vi "fetch frame usb 悉灵.vi"() -> ()   [LabVIEW 2015]
uses:
  <vilib>/Utility/miscctls.llb/LV3DPointTypeDef.ctl
  <vilib>/Utility/miscctls.llb/LVRGBAColorTypeDef.ctl
  <userlib>/Mv3dRgbd/Mv3dRgbd.lvlib
  <vilib>/picture/3D Picture Control/NI_3D Picture Control.lvlib
  <userlib>/Mv3dRgbdEx/Mv3dRgbdEx.lvlib
panel:
  out "handle out 4":u32
  out "pProcess out":u32
  out "function return 6":i32
  in  "pProcess":u32
  out "handle out 3":u32
  out "function return 5":i32
  out "pstParam out":T1={"enParamType"=1, "nReserved[0]"=0, "nReserved[1]"=0, "nReserved[2]"=0, "nReserved[3]"=0, "nReserved[4]"=0, "nReserved[5]"=0, "nReserved[6]"=0, "nReserved[7]"=0, "nReserved[8]"=0, "nReserved[9]"=0, "nReserved[10]"=0, "nReserved[11]"=0, "nReserved[12]"=0, "nReserved[13]"=0, "nReserved[14]"=0, "nReserved[15]"=0} {"enParamType" items=["ParamType_Bool"=1, "ParamType_Int"=2, "ParamType_Float"=3, "ParamType_Enum"=4, "ParamType_String"=5]}
  in  "strKey":string
  in  "pstParam":T1={"enParamType"=1, "nReserved[0]"=0, "nReserved[1]"=0, "nReserved[2]"=0, "nReserved[3]"=0, "nReserved[4]"=0, "nReserved[5]"=0, "nReserved[6]"=0, "nReserved[7]"=0, "nReserved[8]"=0, "nReserved[9]"=0, "nReserved[10]"=0, "nReserved[11]"=0, "nReserved[12]"=0, "nReserved[13]"=0, "nReserved[14]"=0, "nReserved[15]"=0} {"enParamType" items=["ParamType_Bool"=1, "ParamType_Int"=2, "ParamType_Float"=3, "ParamType_Enum"=4, "ParamType_String"=5]}
  out "function return 4":i32
  out "pDeviceNumber out":u32
  in  "pDeviceNumber":u32
  out "handle out":u32
  out "function return 3":i32
  out "pstCalibInfo out":T2
  in  "nCoordinateType":u32
  in  "pstCalibInfo":T2
  out "function return 2":i32
  out "size 3":i32
  out "address 3":i64
  out "pYuvImgge out":T3
  in  "handle":u32
  out "pstU3DeviceInfo out":T4
  out "function return":i32
  out "get list return":i32
  out "pDeviceCount out 2":u32
  out "address 2":i64
  out "size 4":i32
  out "address 5":i64
  in  "?":enum32{"RGBD", "点云"}(tab)
  out "Depth":i16[][](graph)
  out "RGB":picture
  out "start function":i32
  out "stop function":i32
  out "release function":i32
  out "init function":i32
  out "close function":i32
  in  "?":bool
  out "fetchframe function":i32
  out "depthtocloud return":i32
  out "yuv422torgb return":i32
  out "MV3D_RGBD_GigEDEVICE_INFO out 3":T5(array[cluster])
  out "?":refnum<vi>(3d-picture)
  in  "Character Size":sgl=0.5 caption="字符大小"
  out "有效点":i32
  out "handle out 2":u32
  out "pstDepthImage out":T3
  out "fetchframe handle out":u32
  out "close handle out":u32
  out "start handle out":u32
  out "stop handle out":u32
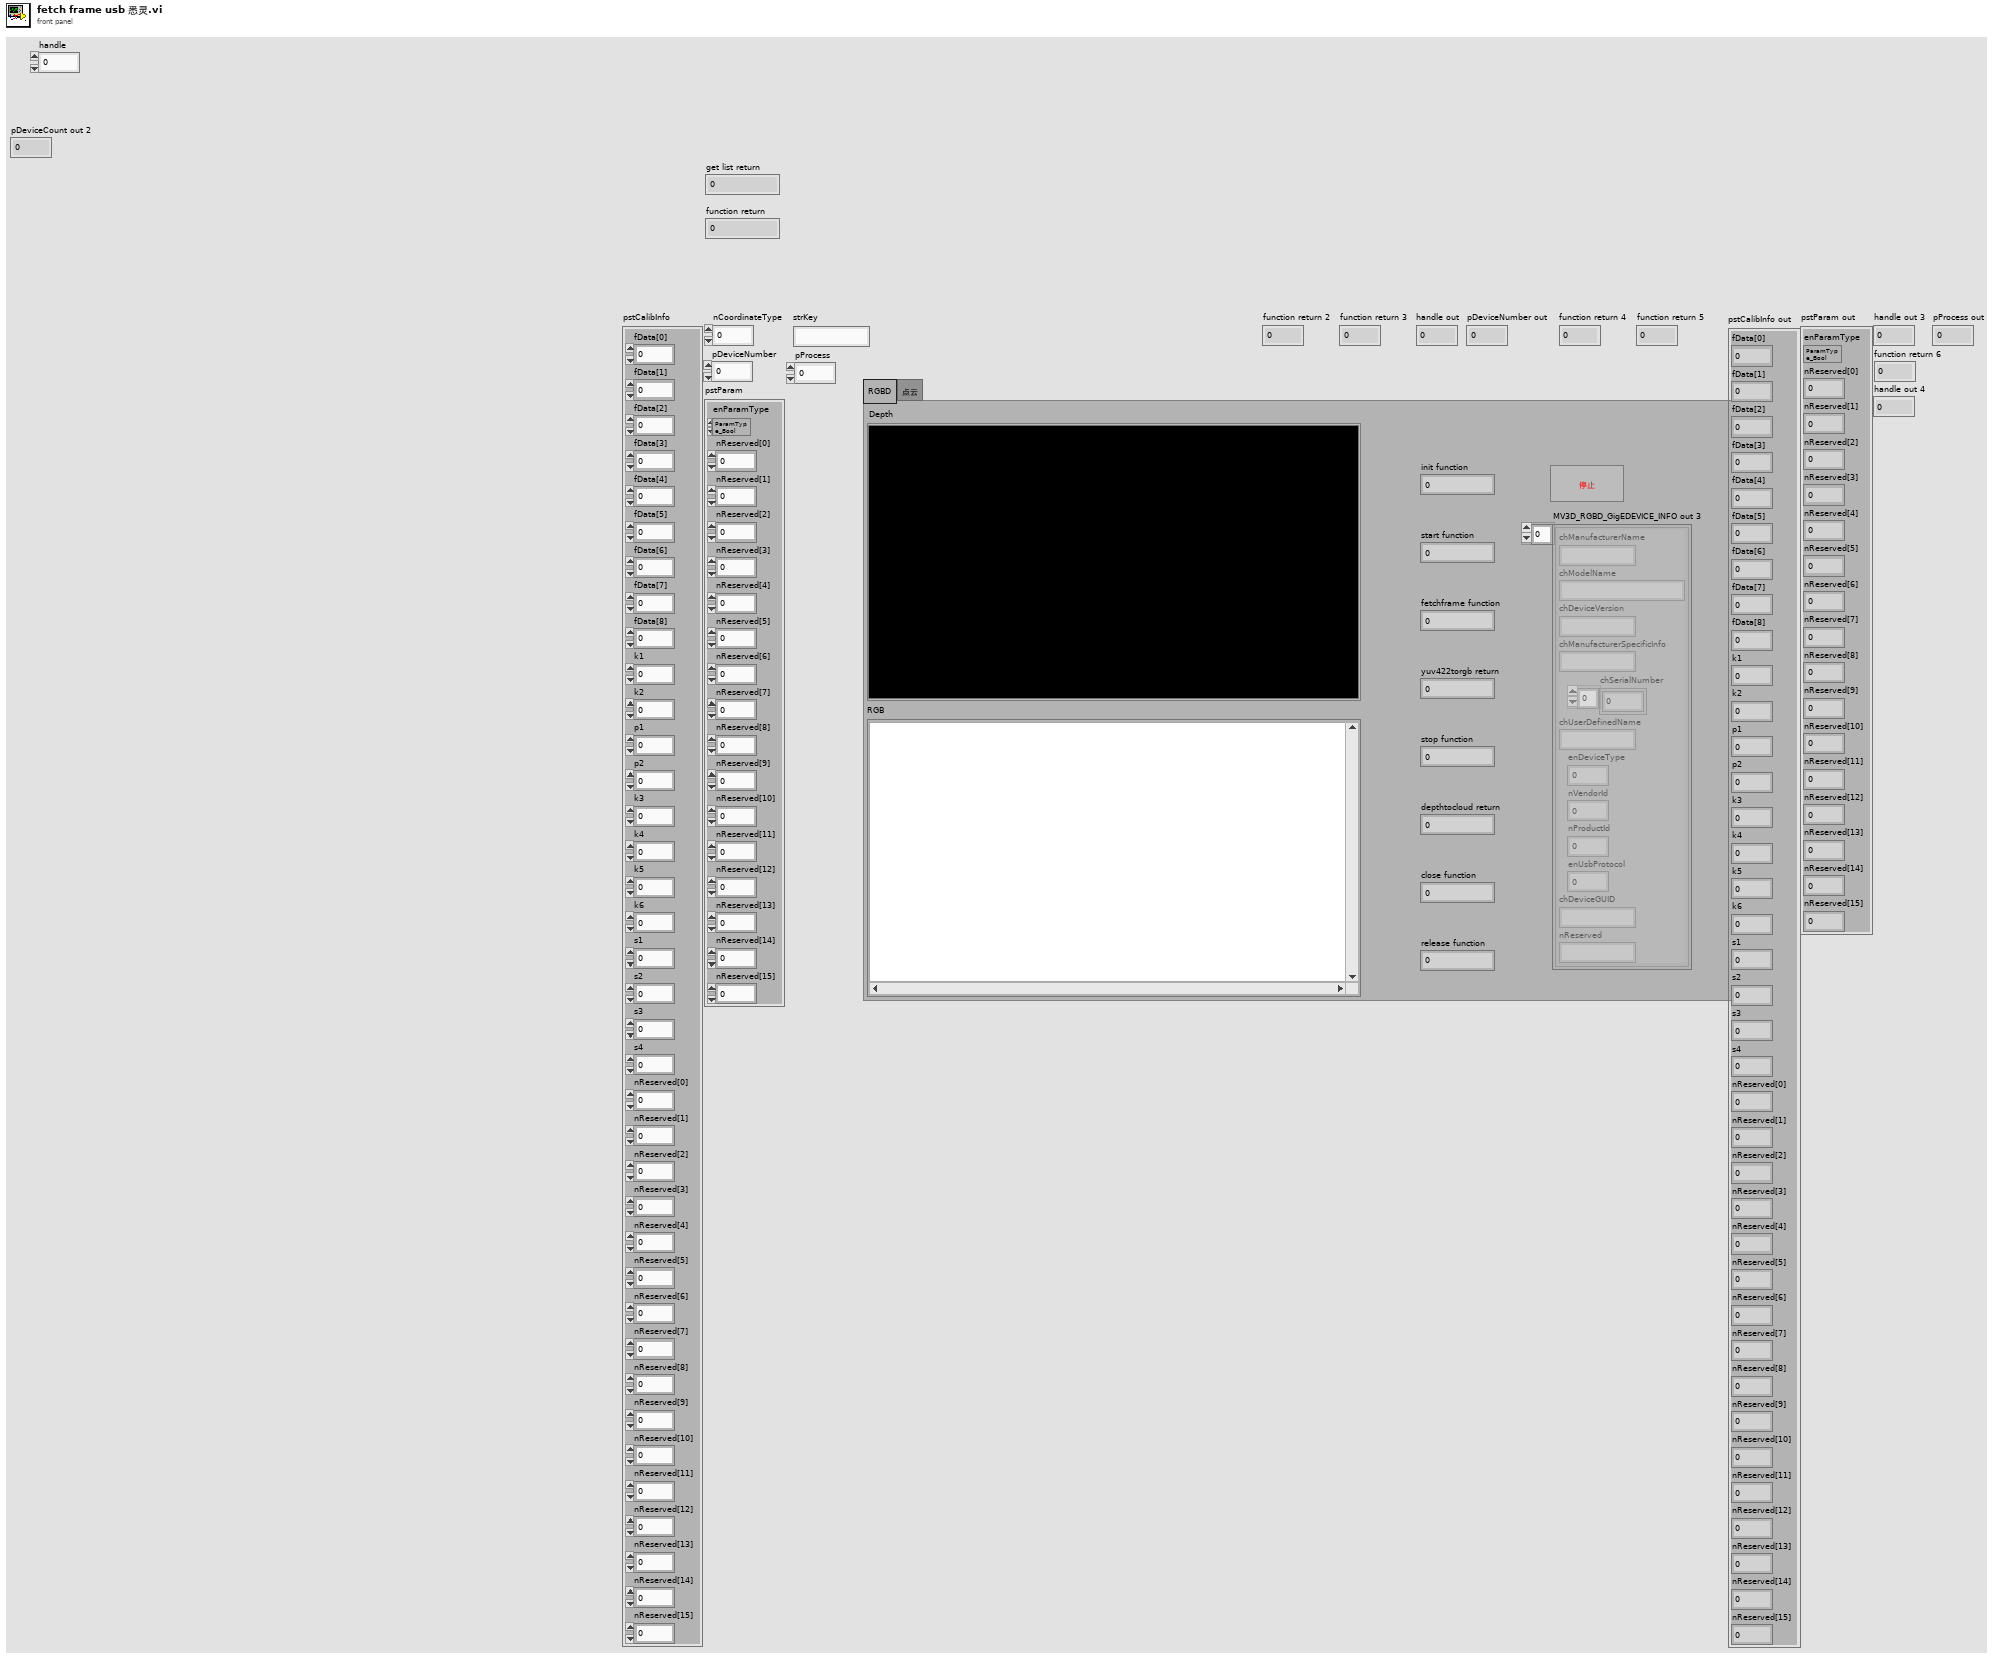
[diagram p1: front panel]
types:
  T1 = cluster{"enParamType":u32, "nReserved[0]":u8, "nReserved[1]":u8, "nReserved[2]":u8, "nReserved[3]":u8, "nReserved[4]":u8, "nReserved[5]":u8, "nReserved[6]":u8, "nReserved[7]":u8, "nReserved[8]":u8, "nReserved[9]":u8, "nReserved[10]":u8, "nReserved[11]":u8, "nReserved[12]":u8, "nReserved[13]":u8, "nReserved[14]":u8, "nReserved[15]":u8}
  T2 = cluster{"fData[0]":sgl, "fData[1]":sgl, "fData[2]":sgl, "fData[3]":sgl, "fData[4]":sgl, "fData[5]":sgl, "fData[6]":sgl, "fData[7]":sgl, "fData[8]":sgl, "k1":sgl, "k2":sgl, "p1":sgl, "p2":sgl, "k3":sgl, "k4":sgl, "k5":sgl, "k6":sgl, "s1":sgl, "s2":sgl, "s3":sgl, "s4":sgl, "nReserved[0]":u8, "nReserved[1]":u8, "nReserved[2]":u8, "nReserved[3]":u8, "nReserved[4]":u8, "nReserved[5]":u8, "nReserved[6]":u8, "nReserved[7]":u8, "nReserved[8]":u8, "nReserved[9]":u8, "nReserved[10]":u8, "nReserved[11]":u8, "nReserved[12]":u8, "nReserved[13]":u8, "nReserved[14]":u8, "nReserved[15]":u8}
  T3 = cluster{"enImageType":i32, "nWidth":u32, "nHeight":u32, "pData":u32, "nDataLen":u32, "nFrameNum":u32, "nTimeStamp":i64, "nReserved[0]":u8, "nReserved[1]":u8, "nReserved[2]":u8, "nReserved[3]":u8, "nReserved[4]":u8, "nReserved[5]":u8, "nReserved[6]":u8, "nReserved[7]":u8, "nReserved[8]":u8, "nReserved[9]":u8, "nReserved[10]":u8, "nReserved[11]":u8, "nReserved[12]":u8, "nReserved[13]":u8, "nReserved[14]":u8, "nReserved[15]":u8}
  T4 = cluster{"chManufacturerName[0]":i8, "chManufacturerName[1]":i8, "chManufacturerName[2]":i8, "chManufacturerName[3]":i8, "chManufacturerName[4]":i8, "chManufacturerName[5]":i8, "chManufacturerName[6]":i8, "chManufacturerName[7]":i8, "chManufacturerName[8]":i8, "chManufacturerName[9]":i8, "chManufacturerName[10]":i8, "chManufacturerName[11]":i8, "chManufacturerName[12]":i8, "chManufacturerName[13]":i8, "chManufacturerName[14]":i8, "chManufacturerName[15]":i8, "chManufacturerName[16]":i8, "chManufacturerName[17]":i8, "chManufacturerName[18]":i8, "chManufacturerName[19]":i8, "chManufacturerName[20]":i8, "chManufacturerName[21]":i8, "chManufacturerName[22]":i8, "chManufacturerName[23]":i8, "chManufacturerName[24]":i8, "chManufacturerName[25]":i8, "chManufacturerName[26]":i8, "chManufacturerName[27]":i8, "chManufacturerName[28]":i8, "chManufacturerName[29]":i8, "chManufacturerName[30]":i8, "chManufacturerName[31]":i8, "chModelName[0]":i8, "chModelName[1]":i8, "chModelName[2]":i8, "chModelName[3]":i8, "chModelName[4]":i8, "chModelName[5]":i8, "chModelName[6]":i8, "chModelName[7]":i8, "chModelName[8]":i8, "chModelName[9]":i8, "chModelName[10]":i8, "chModelName[11]":i8, "chModelName[12]":i8, "chModelName[13]":i8, "chModelName[14]":i8, "chModelName[15]":i8, "chModelName[16]":i8, "chModelName[17]":i8, "chModelName[18]":i8, "chModelName[19]":i8, "chModelName[20]":i8, "chModelName[21]":i8, "chModelName[22]":i8, "chModelName[23]":i8, "chModelName[24]":i8, "chModelName[25]":i8, "chModelName[26]":i8, "chModelName[27]":i8, "chModelName[28]":i8, "chModelName[29]":i8, "chModelName[30]":i8, "chModelName[31]":i8, "chDeviceVersion[0]":i8, "chDeviceVersion[1]":i8, "chDeviceVersion[2]":i8, "chDeviceVersion[3]":i8, "chDeviceVersion[4]":i8, "chDeviceVersion[5]":i8, "chDeviceVersion[6]":i8, "chDeviceVersion[7]":i8, "chDeviceVersion[8]":i8, "chDeviceVersion[9]":i8, "chDeviceVersion[10]":i8, "chDeviceVersion[11]":i8, "chDeviceVersion[12]":i8, "chDeviceVersion[13]":i8, "chDeviceVersion[14]":i8, "chDeviceVersion[15]":i8, "chDeviceVersion[16]":i8, "chDeviceVersion[17]":i8, "chDeviceVersion[18]":i8, "chDeviceVersion[19]":i8, "chDeviceVersion[20]":i8, "chDeviceVersion[21]":i8, "chDeviceVersion[22]":i8, "chDeviceVersion[23]":i8, "chDeviceVersion[24]":i8, "chDeviceVersion[25]":i8, "chDeviceVersion[26]":i8, "chDeviceVersion[27]":i8, "chDeviceVersion[28]":i8, "chDeviceVersion[29]":i8, "chDeviceVersion[30]":i8, "chDeviceVersion[31]":i8, "chManufacturerSpecificInfo[0]":i8, "chManufacturerSpecificInfo[1]":i8, "chManufacturerSpecificInfo[2]":i8, "chManufacturerSpecificInfo[3]":i8, "chManufacturerSpecificInfo[4]":i8, "chManufacturerSpecificInfo[5]":i8, "chManufacturerSpecificInfo[6]":i8, "chManufacturerSpecificInfo[7]":i8, "chManufacturerSpecificInfo[8]":i8, "chManufacturerSpecificInfo[9]":i8, "chManufacturerSpecificInfo[10]":i8, "chManufacturerSpecificInfo[11]":i8, "chManufacturerSpecificInfo[12]":i8, "chManufacturerSpecificInfo[13]":i8, "chManufacturerSpecificInfo[14]":i8, "chManufacturerSpecificInfo[15]":i8, "chManufacturerSpecificInfo[16]":i8, "chManufacturerSpecificInfo[17]":i8, "chManufacturerSpecificInfo[18]":i8, "chManufacturerSpecificInfo[19]":i8, "chManufacturerSpecificInfo[20]":i8, "chManufacturerSpecificInfo[21]":i8, "chManufacturerSpecificInfo[22]":i8, "chManufacturerSpecificInfo[23]":i8, "chManufacturerSpecificInfo[24]":i8, "chManufacturerSpecificInfo[25]":i8, "chManufacturerSpecificInfo[26]":i8, "chManufacturerSpecificInfo[27]":i8, "chManufacturerSpecificInfo[28]":i8, "chManufacturerSpecificInfo[29]":i8, "chManufacturerSpecificInfo[30]":i8, "chManufacturerSpecificInfo[31]":i8, "chManufacturerSpecificInfo[32]":i8, "chManufacturerSpecificInfo[33]":i8, "chManufacturerSpecificInfo[34]":i8, "chManufacturerSpecificInfo[35]":i8, "chManufacturerSpecificInfo[36]":i8, "chManufacturerSpecificInfo[37]":i8, "chManufacturerSpecificInfo[38]":i8, "chManufacturerSpecificInfo[39]":i8, "chManufacturerSpecificInfo[40]":i8, "chManufacturerSpecificInfo[41]":i8, "chManufacturerSpecificInfo[42]":i8, "chManufacturerSpecificInfo[43]":i8, "chManufacturerSpecificInfo[44]":i8, "chManufacturerSpecificInfo[45]":i8, "chManufacturerSpecificInfo[46]":i8, "chManufacturerSpecificInfo[47]":i8, "chSerialNumber[0]":i8, "chSerialNumber[1]":i8, "chSerialNumber[2]":i8, "chSerialNumber[3]":i8, "chSerialNumber[4]":i8, "chSerialNumber[5]":i8, "chSerialNumber[6]":i8, "chSerialNumber[7]":i8, "chSerialNumber[8]":i8, "chSerialNumber[9]":i8, "chSerialNumber[10]":i8, "chSerialNumber[11]":i8, "chSerialNumber[12]":i8, "chSerialNumber[13]":i8, "chSerialNumber[14]":i8, "chSerialNumber[15]":i8, "chUserDefinedName[0]":i8, "chUserDefinedName[1]":i8, "chUserDefinedName[2]":i8, "chUserDefinedName[3]":i8, "chUserDefinedName[4]":i8, "chUserDefinedName[5]":i8, "chUserDefinedName[6]":i8, "chUserDefinedName[7]":i8, "chUserDefinedName[8]":i8, "chUserDefinedName[9]":i8, "chUserDefinedName[10]":i8, "chUserDefinedName[11]":i8, "chUserDefinedName[12]":i8, "chUserDefinedName[13]":i8, "chUserDefinedName[14]":i8, "chUserDefinedName[15]":i8, "enDeviceType":i32, "nVendorId":u32, "nProductId":u32, "enUsbProtocol":i32, "chDeviceGUID[0]":i8, "chDeviceGUID[1]":i8, "chDeviceGUID[2]":i8, "chDeviceGUID[3]":i8, "chDeviceGUID[4]":i8, "chDeviceGUID[5]":i8, "chDeviceGUID[6]":i8, "chDeviceGUID[7]":i8, "chDeviceGUID[8]":i8, "chDeviceGUID[9]":i8, "chDeviceGUID[10]":i8, "chDeviceGUID[11]":i8, "chDeviceGUID[12]":i8, "chDeviceGUID[13]":i8, "chDeviceGUID[14]":i8, "chDeviceGUID[15]":i8, "chDeviceGUID[16]":i8, "chDeviceGUID[17]":i8, "chDeviceGUID[18]":i8, "chDeviceGUID[19]":i8, "chDeviceGUID[20]":i8, "chDeviceGUID[21]":i8, "chDeviceGUID[22]":i8, "chDeviceGUID[23]":i8, "chDeviceGUID[24]":i8, "chDeviceGUID[25]":i8, "chDeviceGUID[26]":i8, "chDeviceGUID[27]":i8, "chDeviceGUID[28]":i8, "chDeviceGUID[29]":i8, "chDeviceGUID[30]":i8, "chDeviceGUID[31]":i8, "chDeviceGUID[32]":i8, "chDeviceGUID[33]":i8, "chDeviceGUID[34]":i8, "chDeviceGUID[35]":i8, "chDeviceGUID[36]":i8, "chDeviceGUID[37]":i8, "chDeviceGUID[38]":i8, "chDeviceGUID[39]":i8, "chDeviceGUID[40]":i8, "chDeviceGUID[41]":i8, "chDeviceGUID[42]":i8, "chDeviceGUID[43]":i8, "chDeviceGUID[44]":i8, "chDeviceGUID[45]":i8, "chDeviceGUID[46]":i8, "chDeviceGUID[47]":i8, "chDeviceGUID[48]":i8, "chDeviceGUID[49]":i8, "chDeviceGUID[50]":i8, "chDeviceGUID[51]":i8, "chDeviceGUID[52]":i8, "chDeviceGUID[53]":i8, "chDeviceGUID[54]":i8, "chDeviceGUID[55]":i8, "chDeviceGUID[56]":i8, "chDeviceGUID[57]":i8, "chDeviceGUID[58]":i8, "chDeviceGUID[59]":i8, "chDeviceGUID[60]":i8, "chDeviceGUID[61]":i8, "chDeviceGUID[62]":i8, "chDeviceGUID[63]":i8, "nReserved[0]":u8, "nReserved[1]":u8, "nReserved[2]":u8, "nReserved[3]":u8, "nReserved[4]":u8, "nReserved[5]":u8, "nReserved[6]":u8, "nReserved[7]":u8, "nReserved[8]":u8, "nReserved[9]":u8, "nReserved[10]":u8, "nReserved[11]":u8, "nReserved[12]":u8, "nReserved[13]":u8, "nReserved[14]":u8, "nReserved[15]":u8}
  T5 = cluster{"chManufacturerName":string, "chModelName":string, "chDeviceVersion":string, "chManufacturerSpecificInfo":string, "chSerialNumber":u8[], "chUserDefinedName":string, "enDeviceType":i32, "nVendorId":u32, "nProductId":u32, "enUsbProtocol":i32, "chDeviceGUID":string, "nReserved":string}[]
  T6 = cluster{"Red":sgl, "Green":sgl, "Blue":sgl, "Alpha":sgl}
  T7 = typedef "LVRGBAColorTypeDef.ctl" = cluster{"Red":sgl, "Green":sgl, "Blue":sgl, "Alpha":sgl}
  T8 = typedef "LV3DPointTypeDef.ctl" = cluster{"X":sgl, "Y":sgl, "Z":sgl}
  T9 = enum16{"Overall", "Per Primitive", "Per Vertex", "Binding Off"}
  T10 = enum16{"Points", "Lines", "Line Strip", "Line Loop", "Triangles", "Triangle Strip", "Triangle Fan", "Quads", "Quad Strip", "Polygon"}
  T11 = cluster{"nImageCount":u64, "MV3D_RGBD_IMAGE_DATA[0]":cluster{"enImageType":i32, "nWidth":u32, "nHeight":u32, "pData":u32, "nDataLen":u32, "nFrameNum":u32, "nTimeStamp":i64, "nReserved[0]":u8, "nReserved[1]":u8, "nReserved[2]":u8, "nReserved[3]":u8, "nReserved[4]":u8, "nReserved[5]":u8, "nReserved[6]":u8, "nReserved[7]":u8, "nReserved[8]":u8, "nReserved[9]":u8, "nReserved[10]":u8, "nReserved[11]":u8, "nReserved[12]":u8, "nReserved[13]":u8, "nReserved[14]":u8, "nReserved[15]":u8}, "MV3D_RGBD_IMAGE_DATA[1]":cluster{"enImageType":i32, "nWidth":u32, "nHeight":u32, "pData":u32, "nDataLen":u32, "nFrameNum":u32, "nTimeStamp":i64, "nReserved[0]":u8, "nReserved[1]":u8, "nReserved[2]":u8, "nReserved[3]":u8, "nReserved[4]":u8, "nReserved[5]":u8, "nReserved[6]":u8, "nReserved[7]":u8, "nReserved[8]":u8, "nReserved[9]":u8, "nReserved[10]":u8, "nReserved[11]":u8, "nReserved[12]":u8, "nReserved[13]":u8, "nReserved[14]":u8, "nReserved[15]":u8}, "MV3D_RGBD_IMAGE_DATA[2]":cluster{"enImageType":i32, "nWidth":u32, "nHeight":u32, "pData":u32, "nDataLen":u32, "nFrameNum":u32, "nTimeStamp":i64, "nReserved[0]":u8, "nReserved[1]":u8, "nReserved[2]":u8, "nReserved[3]":u8, "nReserved[4]":u8, "nReserved[5]":u8, "nReserved[6]":u8, "nReserved[7]":u8, "nReserved[8]":u8, "nReserved[9]":u8, "nReserved[10]":u8, "nReserved[11]":u8, "nReserved[12]":u8, "nReserved[13]":u8, "nReserved[14]":u8, "nReserved[15]":u8}, "MV3D_RGBD_IMAGE_DATA[3]":cluster{"enImageType":i32, "nWidth":u32, "nHeight":u32, "pData":u32, "nDataLen":u32, "nFrameNum":u32, "nTimeStamp":i64, "nReserved[0]":u8, "nReserved[1]":u8, "nReserved[2]":u8, "nReserved[3]":u8, "nReserved[4]":u8, "nReserved[5]":u8, "nReserved[6]":u8, "nReserved[7]":u8, "nReserved[8]":u8, "nReserved[9]":u8, "nReserved[10]":u8, "nReserved[11]":u8, "nReserved[12]":u8, "nReserved[13]":u8, "nReserved[14]":u8, "nReserved[15]":u8}, "MV3D_RGBD_IMAGE_DATA[4]":cluster{"enImageType":i32, "nWidth":u32, "nHeight":u32, "pData":u32, "nDataLen":u32, "nFrameNum":u32, "nTimeStamp":i64, "nReserved[0]":u8, "nReserved[1]":u8, "nReserved[2]":u8, "nReserved[3]":u8, "nReserved[4]":u8, "nReserved[5]":u8, "nReserved[6]":u8, "nReserved[7]":u8, "nReserved[8]":u8, "nReserved[9]":u8, "nReserved[10]":u8, "nReserved[11]":u8, "nReserved[12]":u8, "nReserved[13]":u8, "nReserved[14]":u8, "nReserved[15]":u8}, "MV3D_RGBD_IMAGE_DATA[5]":cluster{"enImageType":i32, "nWidth":u32, "nHeight":u32, "pData":u32, "nDataLen":u32, "nFrameNum":u32, "nTimeStamp":i64, "nReserved[0]":u8, "nReserved[1]":u8, "nReserved[2]":u8, "nReserved[3]":u8, "nReserved[4]":u8, "nReserved[5]":u8, "nReserved[6]":u8, "nReserved[7]":u8, "nReserved[8]":u8, "nReserved[9]":u8, "nReserved[10]":u8, "nReserved[11]":u8, "nReserved[12]":u8, "nReserved[13]":u8, "nReserved[14]":u8, "nReserved[15]":u8}, "MV3D_RGBD_IMAGE_DATA[6]":cluster{"enImageType":i32, "nWidth":u32, "nHeight":u32, "pData":u32, "nDataLen":u32, "nFrameNum":u32, "nTimeStamp":i64, "nReserved[0]":u8, "nReserved[1]":u8, "nReserved[2]":u8, "nReserved[3]":u8, "nReserved[4]":u8, "nReserved[5]":u8, "nReserved[6]":u8, "nReserved[7]":u8, "nReserved[8]":u8, "nReserved[9]":u8, "nReserved[10]":u8, "nReserved[11]":u8, "nReserved[12]":u8, "nReserved[13]":u8, "nReserved[14]":u8, "nReserved[15]":u8}, "MV3D_RGBD_IMAGE_DATA[7]":cluster{"enImageType":i32, "nWidth":u32, "nHeight":u32, "pData":u32, "nDataLen":u32, "nFrameNum":u32, "nTimeStamp":i64, "nReserved[0]":u8, "nReserved[1]":u8, "nReserved[2]":u8, "nReserved[3]":u8, "nReserved[4]":u8, "nReserved[5]":u8, "nReserved[6]":u8, "nReserved[7]":u8, "nReserved[8]":u8, "nReserved[9]":u8, "nReserved[10]":u8, "nReserved[11]":u8, "nReserved[12]":u8, "nReserved[13]":u8, "nReserved[14]":u8, "nReserved[15]":u8}, "MV3D_RGBD_IMAGE_DATA[8]":cluster{"enImageType":i32, "nWidth":u32, "nHeight":u32, "pData":u32, "nDataLen":u32, "nFrameNum":u32, "nTimeStamp":i64, "nReserved[0]":u8, "nReserved[1]":u8, "nReserved[2]":u8, "nReserved[3]":u8, "nReserved[4]":u8, "nReserved[5]":u8, "nReserved[6]":u8, "nReserved[7]":u8, "nReserved[8]":u8, "nReserved[9]":u8, "nReserved[10]":u8, "nReserved[11]":u8, "nReserved[12]":u8, "nReserved[13]":u8, "nReserved[14]":u8, "nReserved[15]":u8}, "MV3D_RGBD_IMAGE_DATA[9]":cluster{"enImageType":i32, "nWidth":u32, "nHeight":u32, "pData":u32, "nDataLen":u32, "nFrameNum":u32, "nTimeStamp":i64, "nReserved[0]":u8, "nReserved[1]":u8, "nReserved[2]":u8, "nReserved[3]":u8, "nReserved[4]":u8, "nReserved[5]":u8, "nReserved[6]":u8, "nReserved[7]":u8, "nReserved[8]":u8, "nReserved[9]":u8, "nReserved[10]":u8, "nReserved[11]":u8, "nReserved[12]":u8, "nReserved[13]":u8, "nReserved[14]":u8, "nReserved[15]":u8}, "nReserved[0]":u8, "nReserved[1]":u8, "nReserved[2]":u8, "nReserved[3]":u8, "nReserved[4]":u8, "nReserved[5]":u8, "nReserved[6]":u8, "nReserved[7]":u8, "nReserved[8]":u8, "nReserved[9]":u8, "nReserved[10]":u8, "nReserved[11]":u8, "nReserved[12]":u8, "nReserved[13]":u8, "nReserved[14]":u8, "nReserved[15]":u8}
  T12 = cluster{"chManufacturerName[0]":i8, "chManufacturerName[1]":i8, "chManufacturerName[2]":i8, "chManufacturerName[3]":i8, "chManufacturerName[4]":i8, "chManufacturerName[5]":i8, "chManufacturerName[6]":i8, "chManufacturerName[7]":i8, "chManufacturerName[8]":i8, "chManufacturerName[9]":i8, "chManufacturerName[10]":i8, "chManufacturerName[11]":i8, "chManufacturerName[12]":i8, "chManufacturerName[13]":i8, "chManufacturerName[14]":i8, "chManufacturerName[15]":i8, "chManufacturerName[16]":i8, "chManufacturerName[17]":i8, "chManufacturerName[18]":i8, "chManufacturerName[19]":i8, "chManufacturerName[20]":i8, "chManufacturerName[21]":i8, "chManufacturerName[22]":i8, "chManufacturerName[23]":i8, "chManufacturerName[24]":i8, "chManufacturerName[25]":i8, "chManufacturerName[26]":i8, "chManufacturerName[27]":i8, "chManufacturerName[28]":i8, "chManufacturerName[29]":i8, "chManufacturerName[30]":i8, "chManufacturerName[31]":i8, "chModelName[0]":i8, "chModelName[1]":i8, "chModelName[2]":i8, "chModelName[3]":i8, "chModelName[4]":i8, "chModelName[5]":i8, "chModelName[6]":i8, "chModelName[7]":i8, "chModelName[8]":i8, "chModelName[9]":i8, "chModelName[10]":i8, "chModelName[11]":i8, "chModelName[12]":i8, "chModelName[13]":i8, "chModelName[14]":i8, "chModelName[15]":i8, "chModelName[16]":i8, "chModelName[17]":i8, "chModelName[18]":i8, "chModelName[19]":i8, "chModelName[20]":i8, "chModelName[21]":i8, "chModelName[22]":i8, "chModelName[23]":i8, "chModelName[24]":i8, "chModelName[25]":i8, "chModelName[26]":i8, "chModelName[27]":i8, "chModelName[28]":i8, "chModelName[29]":i8, "chModelName[30]":i8, "chModelName[31]":i8, "chDeviceVersion[0]":i8, "chDeviceVersion[1]":i8, "chDeviceVersion[2]":i8, "chDeviceVersion[3]":i8, "chDeviceVersion[4]":i8, "chDeviceVersion[5]":i8, "chDeviceVersion[6]":i8, "chDeviceVersion[7]":i8, "chDeviceVersion[8]":i8, "chDeviceVersion[9]":i8, "chDeviceVersion[10]":i8, "chDeviceVersion[11]":i8, "chDeviceVersion[12]":i8, "chDeviceVersion[13]":i8, "chDeviceVersion[14]":i8, "chDeviceVersion[15]":i8, "chDeviceVersion[16]":i8, "chDeviceVersion[17]":i8, "chDeviceVersion[18]":i8, "chDeviceVersion[19]":i8, "chDeviceVersion[20]":i8, "chDeviceVersion[21]":i8, "chDeviceVersion[22]":i8, "chDeviceVersion[23]":i8, "chDeviceVersion[24]":i8, "chDeviceVersion[25]":i8, "chDeviceVersion[26]":i8, "chDeviceVersion[27]":i8, "chDeviceVersion[28]":i8, "chDeviceVersion[29]":i8, "chDeviceVersion[30]":i8, "chDeviceVersion[31]":i8, "chManufacturerSpecificInfo[0]":i8, "chManufacturerSpecificInfo[1]":i8, "chManufacturerSpecificInfo[2]":i8, "chManufacturerSpecificInfo[3]":i8, "chManufacturerSpecificInfo[4]":i8, "chManufacturerSpecificInfo[5]":i8, "chManufacturerSpecificInfo[6]":i8, "chManufacturerSpecificInfo[7]":i8, "chManufacturerSpecificInfo[8]":i8, "chManufacturerSpecificInfo[9]":i8, "chManufacturerSpecificInfo[10]":i8, "chManufacturerSpecificInfo[11]":i8, "chManufacturerSpecificInfo[12]":i8, "chManufacturerSpecificInfo[13]":i8, "chManufacturerSpecificInfo[14]":i8, "chManufacturerSpecificInfo[15]":i8, "chManufacturerSpecificInfo[16]":i8, "chManufacturerSpecificInfo[17]":i8, "chManufacturerSpecificInfo[18]":i8, "chManufacturerSpecificInfo[19]":i8, "chManufacturerSpecificInfo[20]":i8, "chManufacturerSpecificInfo[21]":i8, "chManufacturerSpecificInfo[22]":i8, "chManufacturerSpecificInfo[23]":i8, "chManufacturerSpecificInfo[24]":i8, "chManufacturerSpecificInfo[25]":i8, "chManufacturerSpecificInfo[26]":i8, "chManufacturerSpecificInfo[27]":i8, "chManufacturerSpecificInfo[28]":i8, "chManufacturerSpecificInfo[29]":i8, "chManufacturerSpecificInfo[30]":i8, "chManufacturerSpecificInfo[31]":i8, "chManufacturerSpecificInfo[32]":i8, "chManufacturerSpecificInfo[33]":i8, "chManufacturerSpecificInfo[34]":i8, "chManufacturerSpecificInfo[35]":i8, "chManufacturerSpecificInfo[36]":i8, "chManufacturerSpecificInfo[37]":i8, "chManufacturerSpecificInfo[38]":i8, "chManufacturerSpecificInfo[39]":i8, "chManufacturerSpecificInfo[40]":i8, "chManufacturerSpecificInfo[41]":i8, "chManufacturerSpecificInfo[42]":i8, "chManufacturerSpecificInfo[43]":i8, "chManufacturerSpecificInfo[44]":i8, "chManufacturerSpecificInfo[45]":i8, "chManufacturerSpecificInfo[46]":i8, "chManufacturerSpecificInfo[47]":i8, "chSerialNumber[0]":i8, "chSerialNumber[1]":i8, "chSerialNumber[2]":i8, "chSerialNumber[3]":i8, "chSerialNumber[4]":i8, "chSerialNumber[5]":i8, "chSerialNumber[6]":i8, "chSerialNumber[7]":i8, "chSerialNumber[8]":i8, "chSerialNumber[9]":i8, "chSerialNumber[10]":i8, "chSerialNumber[11]":i8, "chSerialNumber[12]":i8, "chSerialNumber[13]":i8, "chSerialNumber[14]":i8, "chSerialNumber[15]":i8, "chUserDefinedName[0]":i8, "chUserDefinedName[1]":i8, "chUserDefinedName[2]":i8, "chUserDefinedName[3]":i8, "chUserDefinedName[4]":i8, "chUserDefinedName[5]":i8, "chUserDefinedName[6]":i8, "chUserDefinedName[7]":i8, "chUserDefinedName[8]":i8, "chUserDefinedName[9]":i8, "chUserDefinedName[10]":i8, "chUserDefinedName[11]":i8, "chUserDefinedName[12]":i8, "chUserDefinedName[13]":i8, "chUserDefinedName[14]":i8, "chUserDefinedName[15]":i8, "enDeviceType":i32, "nVendorId":u32, "nProductId":u32, "enUsbProtocol":i32, "chDeviceGUID[0]":i8, "chDeviceGUID[1]":i8, "chDeviceGUID[2]":i8, "chDeviceGUID[3]":i8, "chDeviceGUID[4]":i8, "chDeviceGUID[5]":i8, "chDeviceGUID[6]":i8, "chDeviceGUID[7]":i8, "chDeviceGUID[8]":i8, "chDeviceGUID[9]":i8, "chDeviceGUID[10]":i8, "chDeviceGUID[11]":i8, "chDeviceGUID[12]":i8, "chDeviceGUID[13]":i8, "chDeviceGUID[14]":i8, "chDeviceGUID[15]":i8, "chDeviceGUID[16]":i8, "chDeviceGUID[17]":i8, "chDeviceGUID[18]":i8, "chDeviceGUID[19]":i8, "chDeviceGUID[20]":i8, "chDeviceGUID[21]":i8, "chDeviceGUID[22]":i8, "chDeviceGUID[23]":i8, "chDeviceGUID[24]":i8, "chDeviceGUID[25]":i8, "chDeviceGUID[26]":i8, "chDeviceGUID[27]":i8, "chDeviceGUID[28]":i8, "chDeviceGUID[29]":i8, "chDeviceGUID[30]":i8, "chDeviceGUID[31]":i8, "chDeviceGUID[32]":i8, "chDeviceGUID[33]":i8, "chDeviceGUID[34]":i8, "chDeviceGUID[35]":i8, "chDeviceGUID[36]":i8, "chDeviceGUID[37]":i8, "chDeviceGUID[38]":i8, "chDeviceGUID[39]":i8, "chDeviceGUID[40]":i8, "chDeviceGUID[41]":i8, "chDeviceGUID[42]":i8, "chDeviceGUID[43]":i8, "chDeviceGUID[44]":i8, "chDeviceGUID[45]":i8, "chDeviceGUID[46]":i8, "chDeviceGUID[47]":i8, "chDeviceGUID[48]":i8, "chDeviceGUID[49]":i8, "chDeviceGUID[50]":i8, "chDeviceGUID[51]":i8, "chDeviceGUID[52]":i8, "chDeviceGUID[53]":i8, "chDeviceGUID[54]":i8, "chDeviceGUID[55]":i8, "chDeviceGUID[56]":i8, "chDeviceGUID[57]":i8, "chDeviceGUID[58]":i8, "chDeviceGUID[59]":i8, "chDeviceGUID[60]":i8, "chDeviceGUID[61]":i8, "chDeviceGUID[62]":i8, "chDeviceGUID[63]":i8, "nReserved[0]":u8, "nReserved[1]":u8, "nReserved[2]":u8, "nReserved[3]":u8, "nReserved[4]":u8, "nReserved[5]":u8, "nReserved[6]":u8, "nReserved[7]":u8, "nReserved[8]":u8, "nReserved[9]":u8, "nReserved[10]":u8, "nReserved[11]":u8, "nReserved[12]":u8, "nReserved[13]":u8, "nReserved[14]":u8, "nReserved[15]":u8}[]
  T13 = typedef "imagedata.ctl" = cluster{"image type":i32, "image depth":i32, "image":u8[], "mask":u8[], "colors":u32[], "Rectangle":cluster{"left":i16, "top":i16, "right":i16, "bottom":i16}}
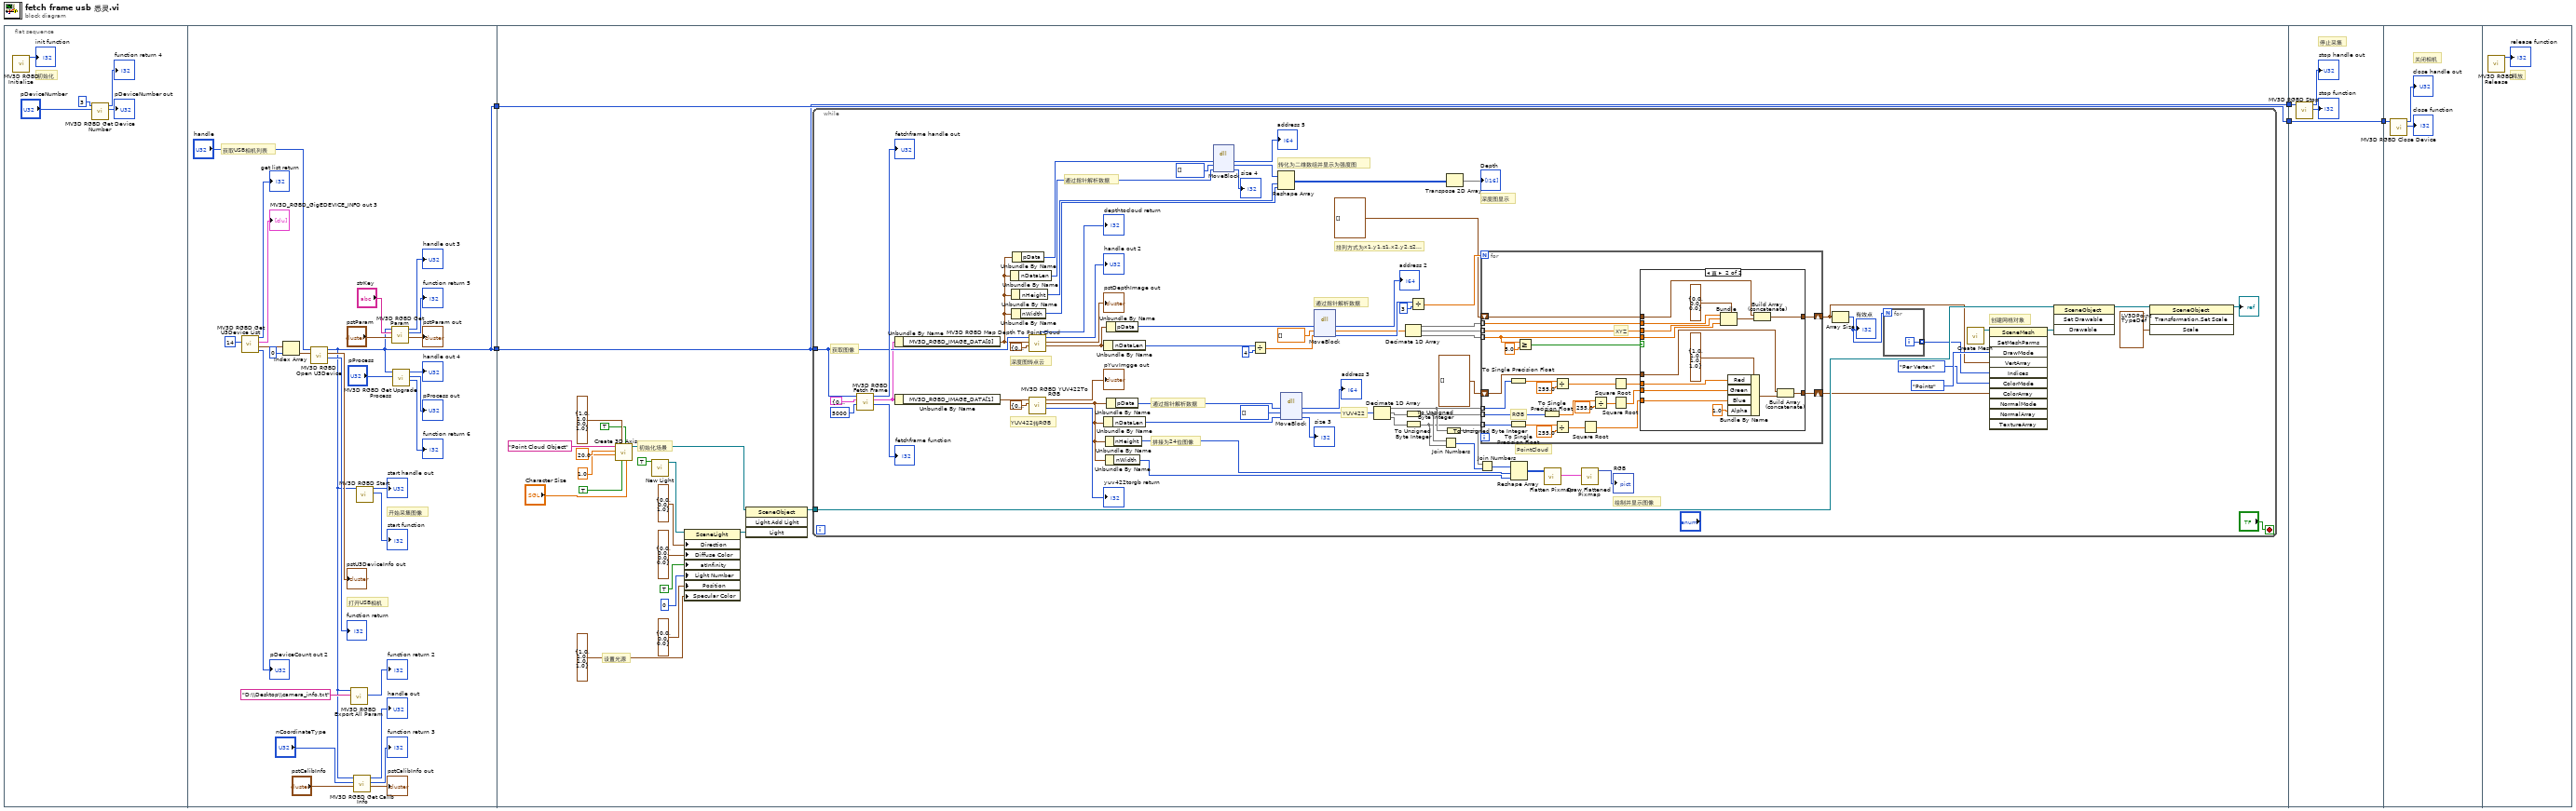
[diagram p0: block diagram]
diagram:
  n1 = flat-sequence {
    tunnel: [w15] -> w2
    tunnel: [w15] -> w1
    tunnel: [w59] -> w4
    tunnel: [w57] -> w3
    tunnel: w2 -> [w57]
    tunnel: w1 -> [w59]
    tunnel: [w176] -> w5
    tunnel: w4 -> [w176]
    tunnel: w3 -> [w177]
    tunnel: w5 -> [w180]
    frame #0 {
      # "初始化"
      n2 = call <userlib>:"MV3D RGBD Initialize.vi"() -> ("function return"=→"init function":i32)  [unwired: 11 in]
      n3 = call <userlib>:"MV3D RGBD Get Device Number.vi"("pDeviceNumber"="pDeviceNumber", "nDeviceType"=u32 3) -> ("pDeviceNumber out"=→"pDeviceNumber out":u32, "function return"=→"function return 4":i32)  [unwired: 8 in]
    }
    frame #1 {
      # "开始采集图像"
      # "打开USB相机"
      # "获取USB相机列表"
      n4 = call <userlib>:"MV3D RGBD Get U3Device List.vi"("nMaxDeviceCount"=u32 14) -> ("pDeviceCount out"=→"pDeviceCount out 2":u32, "MV3D_RGBD_GigEDEVICE_ByteINFO out 2"=w35:T12, "MV3D_RGBD_GigEDEVICE_INFO out 2"=→"MV3D_RGBD_GigEDEVICE_INFO out 3":T5, "function return"=→"get list return":i32)  [unwired: 7 in]
      n5 = Index Array(array=w35, index=0 ("索引")) -> (element=w29:T4)
      n6 = call <userlib>:"MV3D RGBD Open U3Device.vi"("pstU3DeviceInfo"=w29, "handle"="handle") -> ("function return"=→"function return":i32, "pstU3DeviceInfo out"=→"pstU3DeviceInfo out":T4, "handle out"=w15:u32)  [unwired: 7 in]
      n7 = call <userlib>:"MV3D RGBD Export All Param.vi"("pOutFileName"="D:\\Desktop\\camera_info.txt", "handle"=w15) -> ("function return"=→"function return 2":i32)  [unwired: 8 in, 1 out]
      n8 = call <userlib>:"MV3D RGBD Get Calib Info.vi"("pstCalibInfo"="pstCalibInfo", "nCoordinateType"="nCoordinateType", "handle"=w15) -> ("pstCalibInfo out"=→"pstCalibInfo out":T2, "function return"=→"function return 3":i32, "handle out"=→"handle out":u32)  [unwired: 6 in]
      n9 = call <userlib>:"MV3D RGBD Start.vi"("handle"=w15) -> ("function return"=→"start function":i32, "handle out"=→"start handle out":u32)  [unwired: 9 in]
      n10 = call <userlib>:"MV3D RGBD Get Param.vi"("pstParam"="pstParam", "strKey"="strKey", "handle"=w15) -> ("pstParam out"=→"pstParam out":T1, "function return"=→"function return 5":i32, "handle out"=→"handle out 3":u32)  [unwired: 6 in]
      n11 = call <userlib>:"MV3D RGBD Get Upgrade Process.vi"("pProcess"="pProcess", "handle"=w15) -> ("function return"=→"function return 6":i32, "pProcess out"=→"pProcess out":u32, "handle out"=→"handle out 4":u32)  [unwired: 7 in]
    }
    frame #2 {
      # "设置光源"
      # "初始化场景"
      n12 = call <vilib>:"Create 3D Axis.vi"("Character Size"="Character Size", "Half plane?"=TRUE, "Axis label?"=TRUE, "Color"=T6 {"Red"=1.0, "Green"=1.0, "Blue"=0.0, "Alpha"=1.0}, "Radius"=sgl 1.0, "Length"=sgl 20.0, "Name"="Point Cloud Object") -> ("New Object Refnum"=w47:refnum<vi>)  [unwired: 3 in, 1 out]
      n13 = call <vilib>:"New Light.vi"("At Infinity"=TRUE) -> ("New Light Refnum"=w54:refnum<vi>)  [unwired: 9 in, 1 out]
      n14 = property class="SceneLight"(reference=w54, "Direction"=T8 {"X"=0.0, "Y"=0.0, "Z"=1.0} ("方向"), "Diffuse Color"=T7 {"Red"=0.0, "Green"=0.0, "Blue"=0.0, "Alpha"=0.0} ("散射光颜色"), "atInfinity"=TRUE ("位于无穷远处"), "Light Number"=0 ("光源编号"), "Position"=T8 {"X"=0.0, "Y"=0.0, "Z"=0.0} ("位置"), "Specular Color"=T7 {"Red"=1.0, "Green"=1.0, "Blue"=1.0, "Alpha"=1.0} ("反光颜色")) -> (reference out=w56:refnum<vi>)  [unwired: 1 in, 1 out]
      n15 = invoke class="SceneObject" method="Light.Add Light"(reference=w47, "Light"=w56) -> (reference out=w58:refnum<vi>)  [unwired: 2 in, 3 out]
      n16 = while {
        tunnel: w57 -> [w125]
        tunnel: w58 -> [w77]
        stop <- "?" stop-if-true
        # "绘制并显示图像"
        # "创建网格对象"
        # "排列方式为x1,y1,z1,x2,y2,z2..."
        # "深度图显示"
        # "转化为二维数组并显示为强度图"
        # "拼接为24位图像"
        # "通过指针解析数据"
        # "通过指针解析数据"
        # "通过指针解析数据"
        # "YUV422转RGB"
        # "深度图转点云"
        # "获取图像"
        # "YUV422"
        # "PointCloud"
        n17 = call <userlib>:"MV3D RGBD Fetch Frame.vi"("nTimeOut"=u32 5000, "pstFrameData"=T11 {"nImageCount"=0, "MV3D_RGBD_IMAGE_DATA[0]"={"enImageType"=0, "nWidth"=0, "nHeight"=0, "pData"=0, "nDataLen"=0, "nFrameNum"=0, "nTimeStamp"=0, "nReserved[0]"=0, "nReserved[1]"=0, "nReserved[2]"=0, "nReserved[3]"=0, "nReserved[4]"=0, "nReserved[5]"=0, "nReserved[6]"=0, "nReserved[7]"=0, "nReserved[8]"=0, "nReserved[9]"=0, "nReserved[10]"=0, "nReserved[11]"=0, "nReserved[12]"=0, "nReserved[13]"=0, "nReserved[14]"=0, "nReserved[15]"=0}, "MV3D_RGBD_IMAGE_DATA[1]"={"enImageType"=0, "nWidth"=0, "nHeight"=0, "pData"=0, "nDataLen"=0, "nFrameNum"=0, "nTimeStamp"=0, "nReserved[0]"=0, "nReserved[1]"=0, "nReserved[2]"=0, "nReserved[3]"=0, "nReserved[4]"=0, "nReserved[5]"=0, "nReserved[6]"=0, "nReserved[7]"=0, "nReserved[8]"=0, "nReserved[9]"=0, "nReserved[10]"=0, "nReserved[11]"=0, "nReserved[12]"=0, "nReserved[13]"=0, "nReserved[14]"=0, "nReserved[15]"=0}, "MV3D_RGBD_IMAGE_DATA[2]"={"enImageType"=0, "nWidth"=0, "nHeight"=0, "pData"=0, "nDataLen"=0, "nFrameNum"=0, "nTimeStamp"=0, "nReserved[0]"=0, "nReserved[1]"=0, "nReserved[2]"=0, "nReserved[3]"=0, "nReserved[4]"=0, "nReserved[5]"=0, "nReserved[6]"=0, "nReserved[7]"=0, "nReserved[8]"=0, "nReserved[9]"=0, "nReserved[10]"=0, "nReserved[11]"=0, "nReserved[12]"=0, "nReserved[13]"=0, "nReserved[14]"=0, "nReserved[15]"=0}, "MV3D_RGBD_IMAGE_DATA[3]"={"enImageType"=0, "nWidth"=0, "nHeight"=0, "pData"=0, "nDataLen"=0, "nFrameNum"=0, "nTimeStamp"=0, "nReserved[0]"=0, "nReserved[1]"=0, "nReserved[2]"=0, "nReserved[3]"=0, "nReserved[4]"=0, "nReserved[5]"=0, "nReserved[6]"=0, "nReserved[7]"=0, "nReserved[8]"=0, "nReserved[9]"=0, "nReserved[10]"=0, "nReserved[11]"=0, "nReserved[12]"=0, "nReserved[13]"=0, "nReserved[14]"=0, "nReserved[15]"=0}, "MV3D_RGBD_IMAGE_DATA[4]"={"enImageType"=0, "nWidth"=0, "nHeight"=0, "pData"=0, "nDataLen"=0, "nFrameNum"=0, "nTimeStamp"=0, "nReserved[0]"=0, "nReserved[1]"=0, "nReserved[2]"=0, "nReserved[3]"=0, "nReserved[4]"=0, "nReserved[5]"=0, "nReserved[6]"=0, "nReserved[7]"=0, "nReserved[8]"=0, "nReserved[9]"=0, "nReserved[10]"=0, "nReserved[11]"=0, "nReserved[12]"=0, "nReserved[13]"=0, "nReserved[14]"=0, "nReserved[15]"=0}, "MV3D_RGBD_IMAGE_DATA[5]"={"enImageType"=0, "nWidth"=0, "nHeight"=0, "pData"=0, "nDataLen"=0, "nFrameNum"=0, "nTimeStamp"=0, "nReserved[0]"=0, "nReserved[1]"=0, "nReserved[2]"=0, "nReserved[3]"=0, "nReserved[4]"=0, "nReserved[5]"=0, "nReserved[6]"=0, "nReserved[7]"=0, "nReserved[8]"=0, "nReserved[9]"=0, "nReserved[10]"=0, "nReserved[11]"=0, "nReserved[12]"=0, "nReserved[13]"=0, "nReserved[14]"=0, "nReserved[15]"=0}, "MV3D_RGBD_IMAGE_DATA[6]"={"enImageType"=0, "nWidth"=0, "nHeight"=0, "pData"=0, "nDataLen"=0, "nFrameNum"=0, "nTimeStamp"=0, "nReserved[0]"=0, "nReserved[1]"=0, "nReserved[2]"=0, "nReserved[3]"=0, "nReserved[4]"=0, "nReserved[5]"=0, "nReserved[6]"=0, "nReserved[7]"=0, "nReserved[8]"=0, "nReserved[9]"=0, "nReserved[10]"=0, "nReserved[11]"=0, "nReserved[12]"=0, "nReserved[13]"=0, "nReserved[14]"=0, "nReserved[15]"=0}, "MV3D_RGBD_IMAGE_DATA[7]"={"enImageType"=0, "nWidth"=0, "nHeight"=0, "pData"=0, "nDataLen"=0, "nFrameNum"=0, "nTimeStamp"=0, "nReserved[0]"=0, "nReserved[1]"=0, "nReserved[2]"=0, "nReserved[3]"=0, "nReserved[4]"=0, "nReserved[5]"=0, "nReserved[6]"=0, "nReserved[7]"=0, "nReserved[8]"=0, "nReserved[9]"=0, "nReserved[10]"=0, "nReserved[11]"=0, "nReserved[12]"=0, "nReserved[13]"=0, "nReserved[14]"=0, "nReserved[15]"=0}, "MV3D_RGBD_IMAGE_DATA[8]"={"enImageType"=0, "nWidth"=0, "nHeight"=0, "pData"=0, "nDataLen"=0, "nFrameNum"=0, "nTimeStamp"=0, "nReserved[0]"=0, "nReserved[1]"=0, "nReserved[2]"=0, "nReserved[3]"=0, "nReserved[4]"=0, "nReserved[5]"=0, "nReserved[6]"=0, "nReserved[7]"=0, "nReserved[8]"=0, "nReserved[9]"=0, "nReserved[10]"=0, "nReserved[11]"=0, "nReserved[12]"=0, "nReserved[13]"=0, "nReserved[14]"=0, "nReserved[15]"=0}, "MV3D_RGBD_IMAGE_DATA[9]"={"enImageType"=0, "nWidth"=0, "nHeight"=0, "pData"=0, "nDataLen"=0, "nFrameNum"=0, "nTimeStamp"=0, "nReserved[0]"=0, "nReserved[1]"=0, "nReserved[2]"=0, "nReserved[3]"=0, "nReserved[4]"=0, "nReserved[5]"=0, "nReserved[6]"=0, "nReserved[7]"=0, "nReserved[8]"=0, "nReserved[9]"=0, "nReserved[10]"=0, "nReserved[11]"=0, "nReserved[12]"=0, "nReserved[13]"=0, "nReserved[14]"=0, "nReserved[15]"=0}, "nReserved[0]"=0, "nReserved[1]"=0, "nReserved[2]"=0, "nReserved[3]"=0, "nReserved[4]"=0, "nReserved[5]"=0, "nReserved[6]"=0, "nReserved[7]"=0, "nReserved[8]"=0, "nReserved[9]"=0, "nReserved[10]"=0, "nReserved[11]"=0, "nReserved[12]"=0, "nReserved[13]"=0, "nReserved[14]"=0, "nReserved[15]"=0}, "handle"=w125) -> ("function return"=→"fetchframe function":i32, "pstFrameData out"=w123:T11, "handle out"=→"fetchframe handle out":u32)  [unwired: 6 in]
        n18 = Unbundle By Name(w123) -> ("MV3D_RGBD_IMAGE_DATA[0]"=w103:T3)
        n19 = Unbundle By Name(w123) -> ("MV3D_RGBD_IMAGE_DATA[1]"=w78:T3)
        n20 = Unbundle By Name(w103) -> ("nDataLen"=w102:u32)
        n21 = Unbundle By Name(w103) -> ("nHeight"=w80:u32)
        n22 = Unbundle By Name(w103) -> ("nWidth"=w79:u32)
        n23 = Unbundle By Name(w103) -> ("pData"=w101:u32)
        n24 = call <userlib>:"MV3D RGBD Map Depth To Point Cloud.vi"("pstPointCloudImage"=T3 {"enImageType"=0, "nWidth"=0, "nHeight"=0, "pData"=0, "nDataLen"=0, "nFrameNum"=0, "nTimeStamp"=0, "nReserved[0]"=0, "nReserved[1]"=0, "nReserved[2]"=0, "nReserved[3]"=0, "nReserved[4]"=0, "nReserved[5]"=0, "nReserved[6]"=0, "nReserved[7]"=0, "nReserved[8]"=0, "nReserved[9]"=0, "nReserved[10]"=0, "nReserved[11]"=0, "nReserved[12]"=0, "nReserved[13]"=0, "nReserved[14]"=0, "nReserved[15]"=0}, "pstDepthImage"=w103, "handle"=w125) -> ("pstPointCloudImage out"=w112:T3, "pstDepthImage out"=→"pstDepthImage out":T3, "handle out"=→"handle out 2":u32, "function return"=→"depthtocloud return":i32)  [unwired: 5 in]
        n25 = call <userlib>:"MV3D RGBD YUV422To RGB.vi"("pRgbImage"=T3 {"enImageType"=0, "nWidth"=0, "nHeight"=0, "pData"=0, "nDataLen"=0, "nFrameNum"=0, "nTimeStamp"=0, "nReserved[0]"=0, "nReserved[1]"=0, "nReserved[2]"=0, "nReserved[3]"=0, "nReserved[4]"=0, "nReserved[5]"=0, "nReserved[6]"=0, "nReserved[7]"=0, "nReserved[8]"=0, "nReserved[9]"=0, "nReserved[10]"=0, "nReserved[11]"=0, "nReserved[12]"=0, "nReserved[13]"=0, "nReserved[14]"=0, "nReserved[15]"=0}, "pYuvImgge"=w78) -> ("function return"=→"yuv422torgb return":i32, "pRgbImage out"=w82:T3, "pYuvImgge out"=→"pYuvImgge out":T3)  [unwired: 7 in]
        n26 = Unbundle By Name(w112) -> ("nDataLen"=w111:u32)
        n27 = Unbundle By Name(w82) -> ("nDataLen"=w87:u32)
        n28 = Unbundle By Name(w82) -> ("nHeight"=w95:u32)
        n29 = Unbundle By Name(w82) -> ("nWidth"=w94:u32)
        n30 = Unbundle By Name(w112) -> ("pData"=w110:u32)
        n31 = Unbundle By Name(w82) -> ("pData"=w86:u32)
        n32 = dll-call lib="LabVIEW" fn="MoveBlock"("address"=w101, "value"=i16[] [] ("value 6"), "size"=w102) -> ("address"=→"address 5":i64, "value"=w106:i16[], "size"=→"size 4":i32)  [unwired: 4 in, 2 out]
        n33 = Divide(x=w111, y=u32 4) -> (x/y=w116:dbl)
        n34 = Reshape Array(w106, w80, w79) -> (w105:i16[][])
        n35 = dll-call lib="LabVIEW" fn="MoveBlock"("address"=w86, "value"=i16[] [] ("value 5"), "size"=w87) -> ("address"=→"address 3":i64, "value"=w88:u8[], "size"=→"size 3":i32)  [unwired: 4 in, 2 out]
        n36 = dll-call lib="LabVIEW" fn="MoveBlock"("address"=w110, "value"=sgl[] [] ("value 3"), "size"=w116) -> ("address"=→"address 2":u64, "value"=w70:sgl[], "size"=w120:i32)  [unwired: 4 in, 2 out]
        n37 = Decimate 1D Array(w88) -> (w76:u8[], w89:u8[], w90:u8[])
        n38 = Decimate 1D Array(w70) -> (w69:sgl[], w68:sgl[], w67:sgl[])
        n39 = To Unsigned Byte Integer(number=w89) -> (unsigned 8bit integer=w75:u8[])
        n40 = To Unsigned Byte Integer(number=w90) -> (unsigned 8bit integer=w74:u8[])
        n41 = Divide(x=w120, y=3) -> (x/y=w121:dbl)
        n42 = Join Numbers(hi=w75, lo=w74) -> ((hi.lo)=w96:u16[])
        n43 = To Unsigned Byte Integer(number=w76) -> (unsigned 8bit integer=w97:u8[])
        n44 = Transpose 2D Array(2D array=w105) -> (transposed array=→"Depth":i16[][])
        n45 = Join Numbers(hi=w97, lo=w96) -> ((hi.lo)=w91:u32[])
        n46 = for {
          N: w121 -> [_]
          shift-right: [w147] -> w73
          shift-left: T7[] [] ("颜色数组") -> [w146]
          tunnel: w76 -> [w158] mode=indexing
          tunnel: w75 -> [w157] mode=indexing
          tunnel: w74 -> [w156] mode=indexing
          tunnel: w69 -> [w145] mode=indexing
          tunnel: w68 -> [w135] mode=indexing
          tunnel: w67 -> [w144] mode=indexing
          shift-right: [w142] -> w65
          shift-left: cluster{sgl, sgl, sgl}[] [] ("数组") -> [w143]
          # "RGB"
          # "XYZ"
          n47 = To Single Precision Float(number=w158) -> (single precision float=w155:sgl)
          n48 = To Single Precision Float(number=w156) -> (single precision float=w152:sgl)
          n49 = Greater Or Equal?(x=w144, y=sgl 5.0) -> (x >= y?=w148:bool)
          n50 = To Single Precision Float(number=w157) -> (single precision float=w153:sgl)
          n51 = Divide(x=w155, y=sgl 255.0) -> (x/y=w140:sgl)
          n52 = Divide(x=w152, y=sgl 255.0) -> (x/y=w137:sgl)
          n53 = Square Root(x=w137) -> (sqrt(x)=w136:sgl)
          n54 = Divide(x=w153, y=sgl 255.0) -> (x/y=w138:sgl)
          n55 = Square Root(x=w140) -> (sqrt(x)=w141:sgl)
          n56 = Square Root(x=w138) -> (sqrt(x)=w139:sgl)
          n57 = case shown="真" w148 {
            tunnel: [w160 w172] -> w147
            tunnel: w146 -> [w160 w171]
            tunnel: w141 -> [_ w170]
            tunnel: w139 -> [_ w169]
            tunnel: w136 -> [_ w168]
            tunnel: [w159 w167] -> w142
            tunnel: w145 -> [_ w165]
            tunnel: w135 -> [_ w164]
            tunnel: w144 -> [_ w163]
            tunnel: w143 -> [w159 w162]
            frame False {
              # "跳过无效点，加快渲染速度"
            }
            frame True {
              n58 = Bundle(cluster=cluster{sgl, sgl, sgl} {0.0, 0.0, 0.0} ("簇"), w165, w164, w163) -> (w166:cluster{sgl, sgl, sgl})
              n59 = Bundle By Name(cluster=T7 {"Red"=1.0, "Green"=1.0, "Blue"=1.0, "Alpha"=1.0} ("Color"), "Red"=w170, "Green"=w169, "Blue"=w168, "Alpha"=sgl 1.0) -> (w175:T7)
              n60 = Build Array (concatenate)(w162, w166) -> (w167:cluster{sgl, sgl, sgl}[])
              n61 = Build Array (concatenate)(w171, w175) -> (w172:T7[])
            }
          }
        }
        n62 = Reshape Array(w91, w95, w94) -> (w92:u32[][])
        n63 = call <vilib>:"Flatten Pixmap.vi"("24-bit pixmap"=w92) -> ("image data"=w93:T13)  [unwired: 10 in]
        n64 = call <vilib>:"Draw Flattened Pixmap.vi"("image data"=w93) -> ("new picture"=→"RGB":picture)  [unwired: 8 in]
        n65 = Array Size(array=w65) -> (size(s)=w64:i32)
        "有效点" <- w64
        n66 = for {
          N: w64 -> [_]
          tunnel: [w134] -> w63 mode=indexing
          i -> [w134]
        }
        n67 = call <vilib>:"Create Mesh.vi"() -> ("New Mesh Refnum"=w117:refnum<vi>)  [unwired: 10 in, 1 out]
        n68 = invoke class="SceneMesh" method="SetMeshParms"(reference=w117, "DrawMode"=T10."Points" ("绘图模式"), "VertArray"=w65, "Indices"=w63, "ColorMode"=T9."Per Vertex" ("颜色绑定模式"), "ColorArray"=w73) -> (reference out=w71:refnum<vi>)  [unwired: 5 in, 10 out]
        n69 = invoke class="SceneObject" method="Set Drawable"(reference=w77, "Drawable"=w71) -> (reference out=w61:refnum<vi>)  [unwired: 2 in, 3 out]
        n70 = invoke class="SceneObject" method="Transformation.Set Scale"(reference=w61, "Scale"=T8 {"X"=0.005, "Y"=0.005, "Z"=0.005} ("缩放")) -> (reference out=→"?":refnum<vi>)  [unwired: 2 in, 3 out]
      }
    }
    frame #3 {
      # "停止采集"
      n71 = call <userlib>:"MV3D RGBD Stop.vi"("handle"=w177) -> ("function return"=→"stop function":i32, "handle out"=→"stop handle out":u32)  [unwired: 9 in]
    }
    frame #4 {
      # "关闭相机"
      n72 = call <userlib>:"MV3D RGBD Close Device.vi"("handle"=w180) -> ("function return"=→"close function":i32, "handle out"=→"close handle out":u32)  [unwired: 9 in]
    }
    frame #5 {
      # "释放"
      n73 = call <userlib>:"MV3D RGBD Release.vi"() -> ("function return"=→"release function":i32)  [unwired: 11 in]
    }
  }
